vi "trg mode constructor.vi"(11 "trg_mode":T1(ring)) -> (3 "trg_mode out":u8)   [LabVIEW 2021, in "libad4.lvlib"]
doc: "Helper to ease the construction of the trigger mode ID."
uses:
  <userlib>/libad4/libad4.lvlib
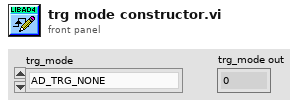
[diagram p1: front panel]
types:
  T1 = enum16{"AD_TRG_NONE", "AD_TRG_POSITIVE", "AD_TRG_NEGATIVE", "AD_TRG_INSIDE", "AD_TRG_OUTSIDE", "AD_TRG_NEVER"}
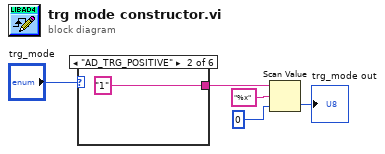
[diagram p0: block diagram]
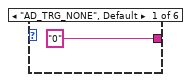
[diagram p2: hidden frame]
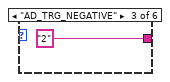
[diagram p3: hidden frame]
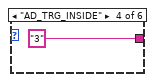
[diagram p4: hidden frame]
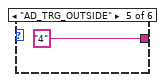
[diagram p5: hidden frame]
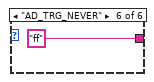
[diagram p6: hidden frame]
diagram:
  n1 = case shown="\"AD_TRG_POSITIVE\"" "trg_mode" {
    tunnel: ["0" "1" "2" "3" "4" "ff"] -> w4
    frame "AD_TRG_NONE", Default {
    }
    frame "AD_TRG_POSITIVE" {
    }
    frame "AD_TRG_NEGATIVE" {
    }
    frame "AD_TRG_INSIDE" {
    }
    frame "AD_TRG_OUTSIDE" {
    }
    frame "AD_TRG_NEVER" {
    }
  }
  n2 = Scan Value(string=w4, format string="%x", default (0 dbl)=u8 0) -> (value=→"trg_mode out":u8)  [unwired: 1 out]
